vi "Initialize Drone index.vi"(8 "error in (no error)":errorcluster, 11 "Reset":bool) -> (0 "error out":errorcluster, 3 "Numeric":i32)   [LabVIEW 2014]
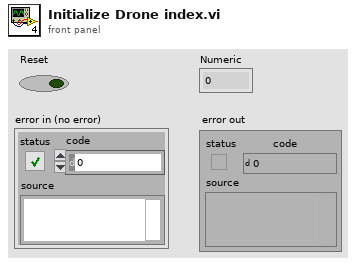
[diagram p1: front panel]
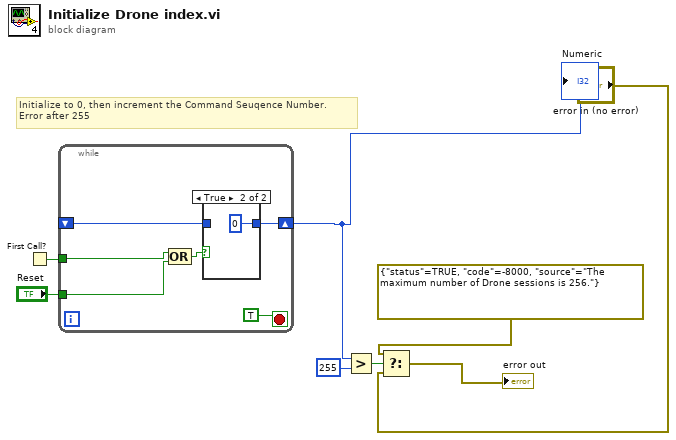
[diagram p0: block diagram]
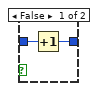
[diagram p2: hidden frame]
diagram:
  # "Initialize to 0, then increment the Command Seuqence Number.\nError after 255"
  n1 = First Call?() -> (First Call?: T/F=w1:bool)
  n2 = while {
    tunnel: w1 -> [w10]
    shift-right: [w13] -> w8
    shift-left: _ -> [w12]
    tunnel: "Reset" -> [w9]
    stop <- TRUE stop-if-true
    n3 = Compound Arithmetic op=OR(w10, w9) -> (w11:bool)
    n4 = case shown="True" w11 {
      tunnel: [w15 0] -> w13
      tunnel: w12 -> [w16 _]
      frame False {
        n5 = Increment(x=w16) -> (x+1=w15:i32)
      }
      frame True {
      }
    }
  }
  "Numeric" <- w8
  n6 = Greater?(x=w8, y=255) -> (0:w4:bool)
  n7 = Select(t=errorcluster {"status"=TRUE, "code"=-8000, "source"="The maximum number of Drone sessions is 256."}, s=w4, f="error in (no error)") -> (s? t:f=→"error out":errorcluster)
